vi "View Phase.vi"(2 "convert to degree (F)":bool, 3 "unwrap phase (F)":bool, 4 "phase (radian)":dbl[](array[numeric]) format="%.2f") -> (0 "unit label (phase)":string, 1 "scaled phase":dbl[](array[numeric]) format="%.2f")   [LabVIEW 2017]
uses:
  <vilib>/Analysis/NI_AALPro.lvlib
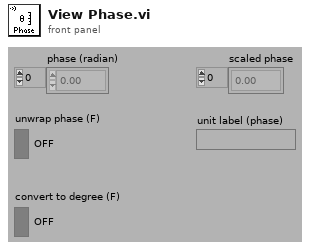
[diagram p1: front panel]
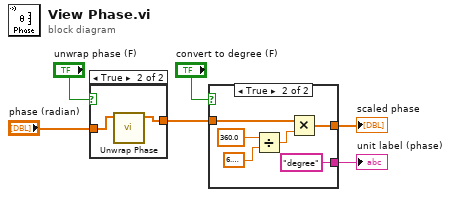
[diagram p0: block diagram]
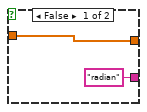
[diagram p3: hidden frame]
diagram:
  n1 = case shown="True" "unwrap phase (F)" {
    tunnel: "phase (radian)" -> [w7 w9]
    tunnel: [w7 w8] -> w2
    frame False {
    }
    frame True {
      n2 = call <vilib>:"Unwrap Phase.vi"("Phase"=w9) -> ("Unwrapped Phase"=w8:dbl[])  [unwired: 9 in, 1 out]
    }
  }
  n3 = case shown="True" "convert to degree (F)" {
    tunnel: [w11 w16] -> w5
    tunnel: w2 -> [w11 w17]
    tunnel: ["radian" ("unit label (phase)") "degree" ("unit label (phase)")] -> w6
    frame False {
    }
    frame True {
      n4 = Divide(x=360.0, y=6.283185307179586) -> (x/y=w12:dbl)
      n5 = Multiply(x=w17, y=w12) -> (x*y=w16:dbl[])
    }
  }
  "unit label (phase)" <- w6
  "scaled phase" <- w5
